vi "PWM Command_TSFTS2.vi"(8 "error in (no error)":errorcluster, 9 "Duty Cycle":i32 min=0 max=100, 10 "Leg":i32 min=0 max=6, 11 "VISA Refnum in":refnum<visa-resource-name>) -> (0 "error out":errorcluster, 2 "Duty Cycle VISA Write":string, 3 "VISA Refnum out":refnum<visa-resource-name>)   [LabVIEW 2022 SP3]
panel:
  out "return count":u32
  out "read buffer":string
  out "Set Duty Cycle":string
  out ">":string
  out "Set PWM Leg":string
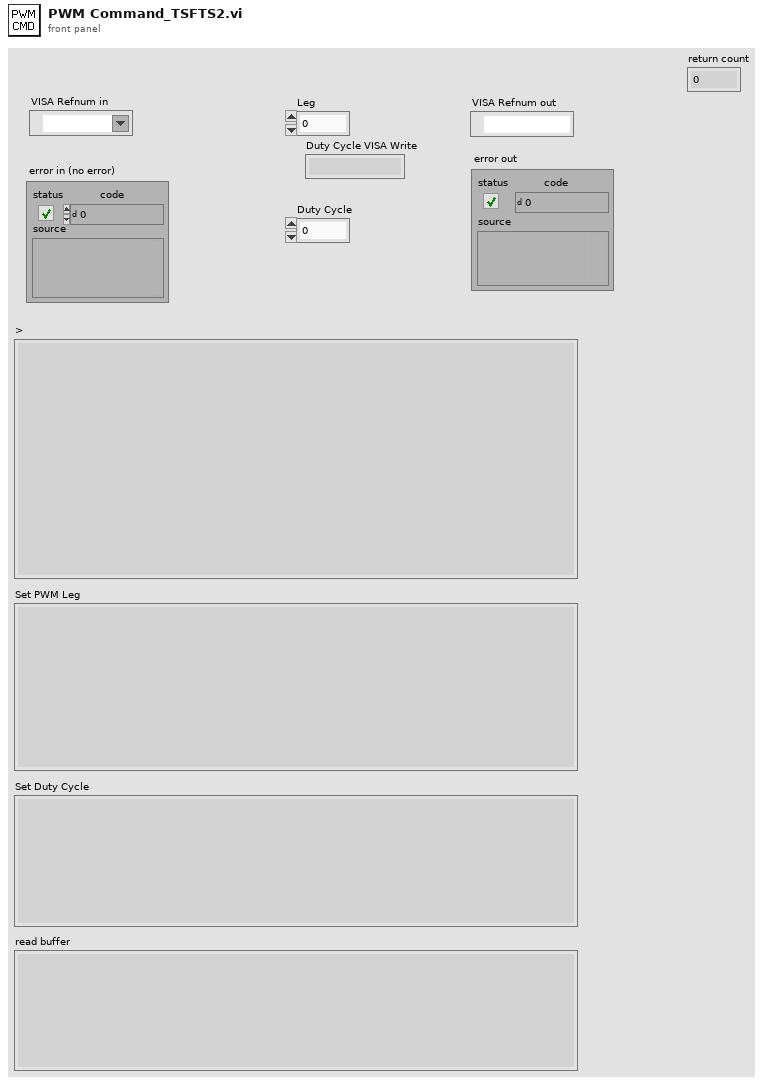
[diagram p1: front panel]
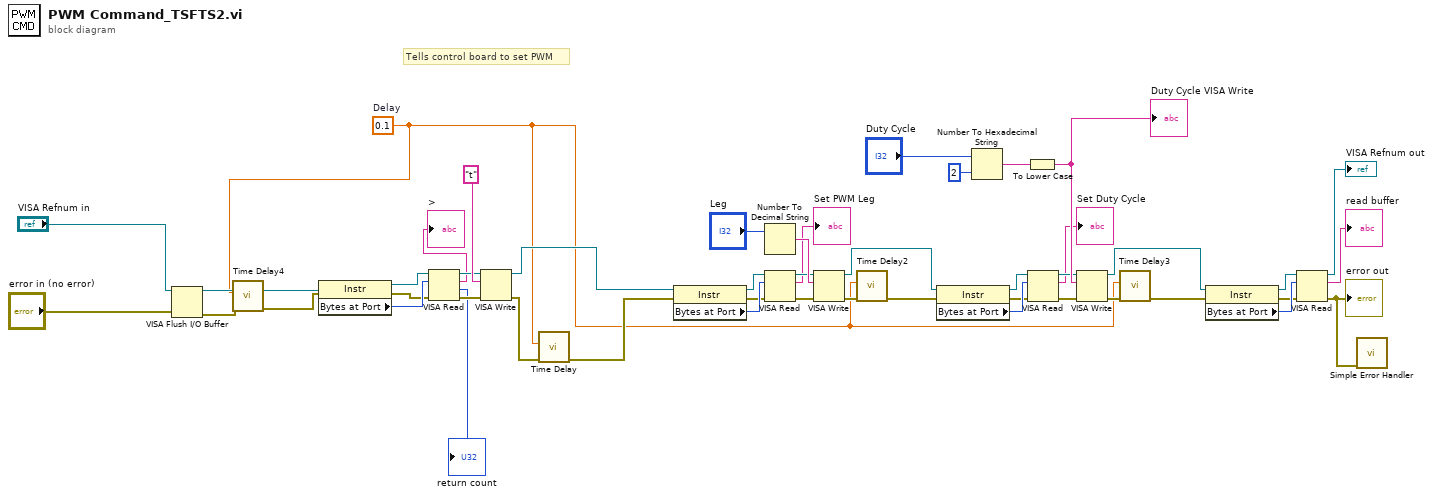
[diagram p0: block diagram]
diagram:
  w1 = 0.1  # Delay
  # "Tells control board to set PWM"
  n1 = VISA Flush I/O Buffer(VISA resource name="VISA Refnum in", error in (no error)="error in (no error)") -> (VISA resource name out=w6:refnum<visa-resource-name>, error out=w3:errorcluster)  [unwired: 1 in]
  n2 = call "Time Delay4"("error in (no error)"=w3, "Delay Time (s)"=w1) -> ("error out"=w2:errorcluster)  [unwired: 9 in]
  n3 = property class="Instr"(reference=w6, error in=w2) -> (reference out=w28:refnum<visa-resource-name>, error out=w8:errorcluster, "Bytes at Port"=w27:u32)
  n4 = VISA Read(VISA resource name=w28, byte count=w27, error in (no error)=w8) -> (VISA resource name out=w29:refnum<visa-resource-name>, read buffer=→">":string, return count=→"return count":u32, error out=w30:errorcluster)
  n5 = VISA Write(VISA resource name=w29, write buffer="t", error in (no error)=w30) -> (VISA resource name out=w42:refnum<visa-resource-name>, error out=w47:errorcluster)  [unwired: 1 out]
  n6 = call "Time Delay"("error in (no error)"=w47, "Delay Time (s)"=w1) -> ("error out"=w25:errorcluster)  [unwired: 9 in]
  n7 = property class="Instr"(reference=w42, error in=w25) -> (reference out=w33:refnum<visa-resource-name>, error out=w24:errorcluster, "Bytes at Port"=w32:u32)
  n8 = Number To Decimal String(number="Leg") -> (decimal integer string=w36:string)  [unwired: 1 in]
  n9 = VISA Read(VISA resource name=w33, byte count=w32, error in (no error)=w24) -> (VISA resource name out=w35:refnum<visa-resource-name>, read buffer=→"Set PWM Leg":string, error out=w34:errorcluster)  [unwired: 1 out]
  n10 = VISA Write(VISA resource name=w35, write buffer=w36, error in (no error)=w34) -> (VISA resource name out=w41:refnum<visa-resource-name>, error out=w40:errorcluster)  [unwired: 1 out]
  n11 = call "Time Delay2"("error in (no error)"=w40, "Delay Time (s)"=w1) -> ("error out"=w18:errorcluster)  [unwired: 9 in]
  n12 = property class="Instr"(reference=w41, error in=w18) -> (reference out=w22:refnum<visa-resource-name>, error out=w19:errorcluster, "Bytes at Port"=w21:u32)
  n13 = Number To Hexadecimal String(1:i16 2 ("width (-)"), 2:"Duty Cycle") -> (0:w44:string)
  n14 = To Lower Case(string=w44) -> (all lower case string=w43:string)
  "Duty Cycle VISA Write" <- w43
  n15 = VISA Read(VISA resource name=w22, byte count=w21, error in (no error)=w19) -> (VISA resource name out=w23:refnum<visa-resource-name>, read buffer=→"Set Duty Cycle":string, error out=w17:errorcluster)  [unwired: 1 out]
  n16 = VISA Write(VISA resource name=w23, write buffer=w43, error in (no error)=w17) -> (VISA resource name out=w45:refnum<visa-resource-name>, error out=w39:errorcluster)  [unwired: 1 out]
  n17 = call "Time Delay3"("error in (no error)"=w39, "Delay Time (s)"=w1) -> ("error out"=w12:errorcluster)  [unwired: 9 in]
  n18 = property class="Instr"(reference=w45, error in=w12) -> (reference out=w15:refnum<visa-resource-name>, error out=w11:errorcluster, "Bytes at Port"=w14:u32)
  n19 = VISA Read(VISA resource name=w15, byte count=w14, error in (no error)=w11) -> (VISA resource name out=→"VISA Refnum out":refnum<visa-resource-name>, read buffer=→"read buffer":string, error out=w9:errorcluster)  [unwired: 1 out]
  "error out" <- w9
  n20 = call <vilib>:"Simple Error Handler.vi"("error in (no error)"=w9) -> ()  [unwired: 4 in, 5 out]
